vi "unpublish event.vi"(7 "module ID":string, 8 "error in":errorcluster, 10 "published element":string, 11 "engine configuration in":refnum<class "engine configuration.lvclass">) -> (0 "error out":errorcluster, 3 "engine configuration out":refnum<class "engine configuration.lvclass">)   [LabVIEW 2013, in "engine configuration.lvclass"]
uses:
  engine configuration.lvclass
  engine configuration.lvclass/engine configuration.ctl
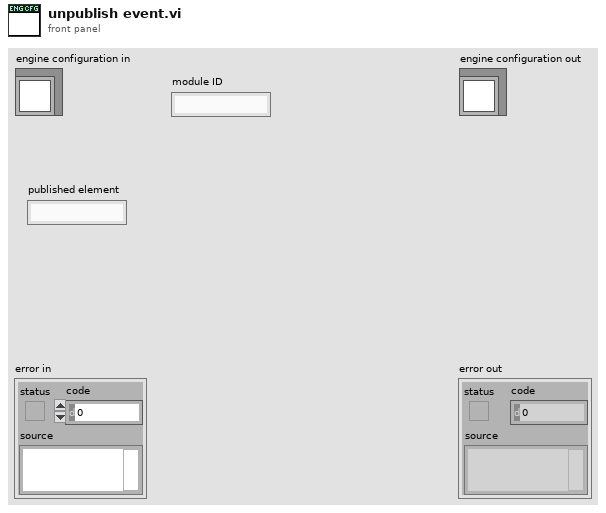
[diagram p1: front panel]
types:
  T1 = typedef "engine configuration.lvclass/simple mapping.ctl" = cluster{"module ID":string[], "publisher":string[], "subscribers":T2[]}
  T2 = typedef "engine configuration.lvclass/module channel pairings.ctl" = cluster{"modules":string[], "element":string[]}
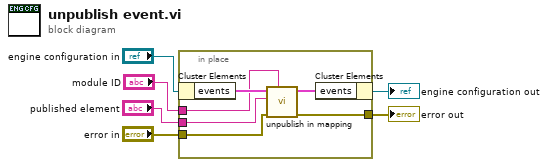
[diagram p0: block diagram]
diagram:
  n1 = in-place {
    in-place-border: "error in" -> [w9]
    in-place-border: "module ID" -> [w7]
    in-place-border: "published element" -> [w11]
    in-place-border: [w10] -> w1
    n2 = in-place-cluster #1("engine configuration in") -> ("events"=w8:T1)
    n3 = call "unpublish in mapping.vi"("module ID"=w7, "error in"=w9, "published element"=w11, "mappings in"=w8) -> ("error out"=w10:errorcluster, "mappings out"=w12:T1)  [unwired: 6 in]
    n4 = in-place-cluster #1("events"=w12) -> (→"engine configuration out":refnum<class "engine configuration.lvclass">)
  }
  "error out" <- w1
